vi "Komponente mit autorange ermitteln.vi"(7 "autorange":bool=TRUE, 10 "Indizes":i32[](array[numeric]), 11 "Gasliste":string[](array[string])) -> (2 "Index":i32, 3 "Gaskomponente":string)   [LabVIEW 2020, in "System Einstellungen V2.lvlib"]
uses:
  System Einstellungen V2.lvlib
  <vilib>/regexp/Match Regular Expression.xnode
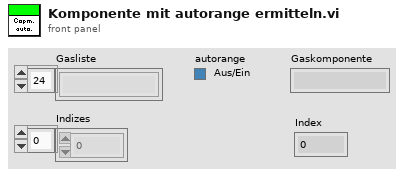
[diagram p1: front panel]
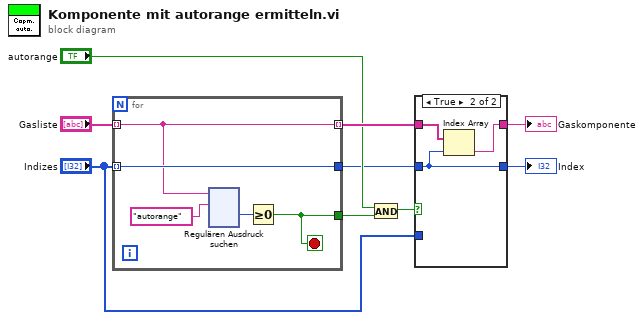
[diagram p0: block diagram]
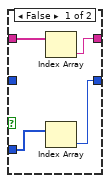
[diagram p2: hidden frame]
diagram:
  n1 = for {
    tunnel: "Gasliste" -> [w10] mode=indexing
    tunnel: "Indizes" -> [w12] mode=indexing
    tunnel: [w12] -> w1
    tunnel: [w11] -> w8
    tunnel: [w10] -> w6 mode=indexing
    stop <- w11 stop-if-true
    n2 = xnode "Regulären Ausdruck suchen"("Eingangs-String"=w10, "Regulärer Ausdruck"="autorange") -> ("Offset nach Übereinstimmung"=w13:i32)  [unwired: 4 in, 4 out]
    n3 = Greater Or Equal To 0?(x=w13) -> (x >= 0?=w11:bool)
  }
  n4 = And(x="autorange", y=w8) -> (x .and. y?=w4:bool)
  n5 = case shown="True" w4 {
    tunnel: "Indizes" -> [w130 _]
    tunnel: w1 -> [_ w133]
    tunnel: [w129 w133] -> w7
    tunnel: w6 -> [w132 w135]
    tunnel: [w131 w134] -> w5
    frame False {
      n6 = Index Array(array=w132) -> (element=w131:string)  [unwired: 1 in]
      n7 = Index Array(array=w130) -> (element=w129:i32)  [unwired: 1 in]
    }
    frame True {
      n8 = Index Array(array=w135, index=w133) -> (element=w134:string)
    }
  }
  "Index" <- w7
  "Gaskomponente" <- w5
